vi "Get_File.vi"(8 "error in (no error)":errorcluster, 11 "IB_Source_File in":refnum<class "IB_Source_File.lvclass">) -> (0 "error out":errorcluster, 2 "data":T1, 3 "IB_Source_File out":refnum<class "IB_Source_File.lvclass">)   [LabVIEW 2020, in "IB_Source_File.lvclass"]
uses:
  <vilib>/AppBuilder/IB_Classes/Source/File/IB_Source_File.lvclass
  <vilib>/AppBuilder/IB_Classes/Source/File/IB_Source_File.lvclass/IB_Source_File.ctl
  <vilib>/AppBuilder/IB_Classes/Shortcut/IB_Shortcut.lvclass
  <vilib>/AppBuilder/IB_Classes/Source/File/IB_Source_File.ctl
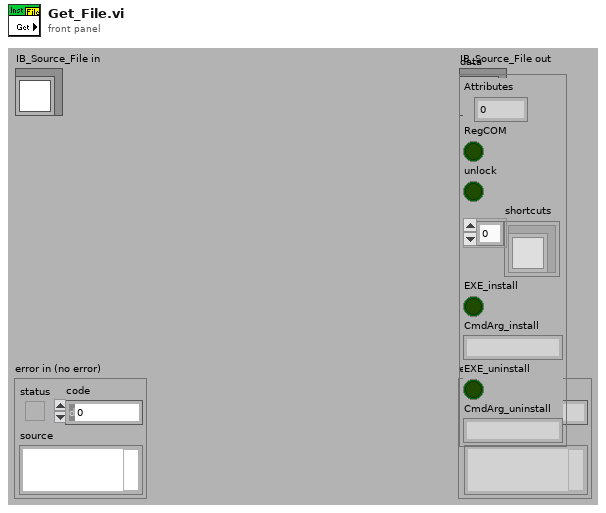
[diagram p1: front panel]
types:
  T1 = typedef "IB_Source_File.ctl" = cluster{"Attributes":i16, "RegCOM":bool, "unlock":bool, "shortcuts":refnum<class "IB_Shortcut.lvclass">[], "EXE_install":bool, "CmdArg_install":string, "EXE_uninstall":bool, "CmdArg_uninstall":string}
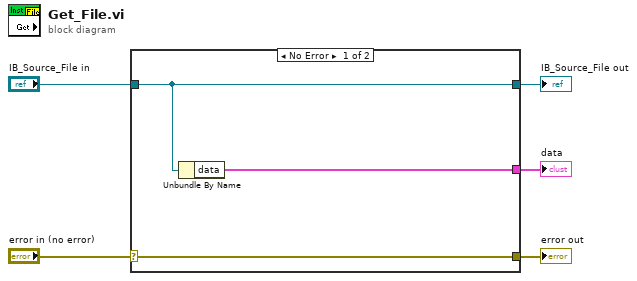
[diagram p0: block diagram]
diagram:
  n1 = case shown="No Error" "error in (no error)" {
    selector: "error in (no error)" -> [w8 w9]
    tunnel: [w8 w9] -> w4
    tunnel: [w7 w10] -> w2
    tunnel: "IB_Source_File in" -> [w7 w10]
    tunnel: [w6 _] -> w1
    frame No Error {
      n2 = Unbundle By Name(w7) -> ("data"=w6:T1)
    }
    frame Error {
    }
  }
  "error out" <- w4
  "IB_Source_File out" <- w2
  "data" <- w1
